vi "SetMenuTagChecked.vi"(8 "error in (no error)":errorcluster, 9 "Checked":bool, 10 "TAG":string, 11 "Gviewer in":refnum<class "Gviewer.lvclass">) -> (0 "error out":errorcluster, 3 "Gviewer out":refnum<class "Gviewer.lvclass">)   [LabVIEW 2020, in "Sgraph_lib_V1.lvlib" / "Gviewer.lvclass"]
doc: "Set Check/Uncheck of one menu item"
uses:
  Gviewer.lvclass
  Gviewer.lvclass/Gviewer.ctl
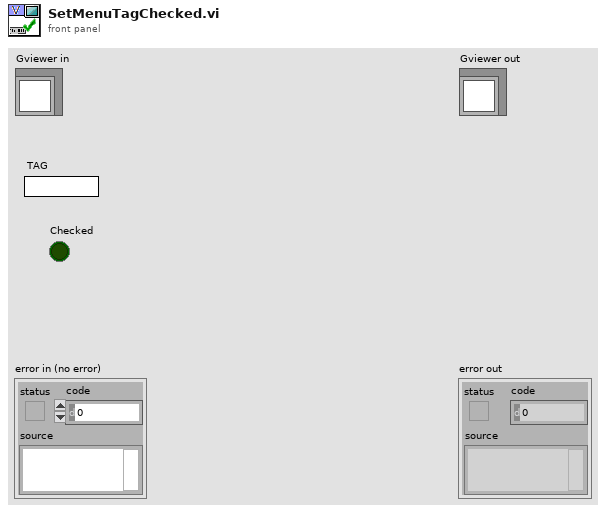
[diagram p1: front panel]
types:
  T1 = typedef "MenuStructure.ctl" = cluster{"After_tag":string, "MenuItems":T2[]}[]
  T2 = typedef "MenuItem.ctl" = cluster{"name":string, "tag":string, "checked":bool, "enabled":bool}
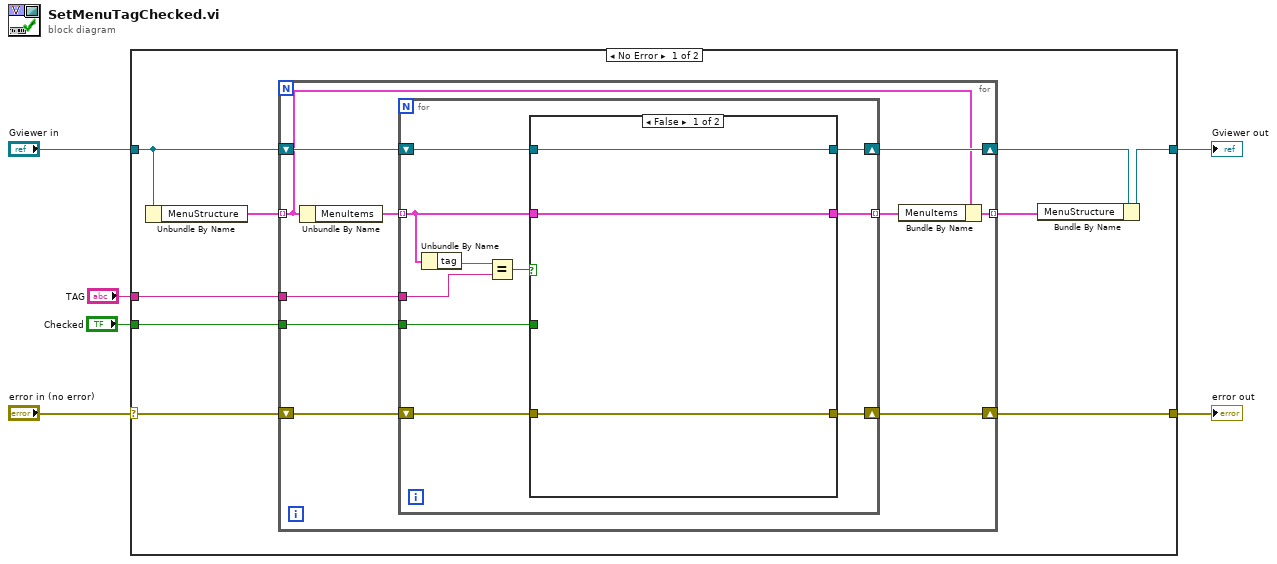
[diagram p0: block diagram]
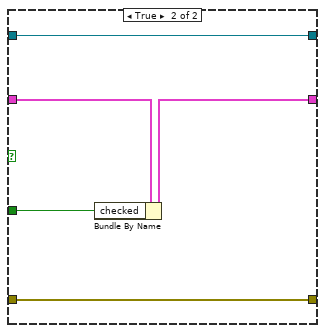
[diagram p2: hidden frame]
diagram:
  n1 = case shown="No Error" "error in (no error)" {
    selector: "error in (no error)" -> [w14 w45]
    tunnel: [w11 w45] -> w5
    tunnel: [w8 w44] -> w3
    tunnel: "Gviewer in" -> [w13 w44]
    tunnel: "TAG" -> [w12 _]
    tunnel: "Checked" -> [w10 _]
    frame No Error {
      n2 = Unbundle By Name(w13) -> ("MenuStructure"=w15:T1)
      n3 = for {
        tunnel: w15 -> [w16] mode=indexing
        tunnel: w12 -> [w24]
        shift-right: [w21] -> w9
        shift-left: w13 -> [w23]
        shift-right: [w20] -> w11
        shift-left: w14 -> [w22]
        tunnel: w10 -> [w19]
        tunnel: [w17] -> w7 mode=indexing
        n4 = Unbundle By Name(w16) -> ("MenuItems"=w25:T2[])
        n5 = for {
          tunnel: w25 -> [w28] mode=indexing
          tunnel: w24 -> [w34]
          shift-right: [w31] -> w21
          shift-left: w23 -> [w32]
          shift-right: [w29] -> w20
          shift-left: w22 -> [w30]
          tunnel: w19 -> [w27]
          tunnel: [w26] -> w18 mode=indexing
          n6 = Unbundle By Name(w28) -> ("tag"=w35:string)
          n7 = Equal?(x=w35, y=w34) -> (x = y?=w33:bool)
          n8 = case shown="False" w33 {
            tunnel: w32 -> [w38 w40]
            tunnel: [w38 w40] -> w31
            tunnel: w30 -> [w37 w39]
            tunnel: [w37 w39] -> w29
            tunnel: w28 -> [w36 w43]
            tunnel: w27 -> [_ w42]
            tunnel: [w36 w41] -> w26
            frame False {
            }
            frame True {
              n9 = Bundle By Name(cluster=w43, "checked"=w42) -> (w41:T2)
            }
          }
        }
        n10 = Bundle By Name(cluster=w16, "MenuItems"=w18) -> (w17:cluster{"After_tag":string, "MenuItems":T2[]})
      }
      n11 = Bundle By Name(cluster=w9, "MenuStructure"=w7) -> (w8:refnum<class "Gviewer.lvclass">)
    }
    frame Error {
    }
  }
  "error out" <- w5
  "Gviewer out" <- w3
